vi "电流传感器测试.vi"(0 "仪器实例 out":T1, 1 "电流读取":refnum<visa-resource-name>, 2 "灵敏度":dbl, 5 "传感器缩放系数":dbl=2000.0 format="%#_13g", 9 "CAB500":enum16{"CAB500", "CAB1500"}(ring), 11 "错误输入（无错误）":errorcluster, 12 "file path (dialog if empty)":path caption="文件路径 （空时为对话框）", 14 "电压读取":bool) -> (3 "报文":string[](array[string]), 4 "仪器实例 out 2":T1, 6 "解析电流":dbl[](array[numeric]), 7 "实读电流":dbl[](array[numeric]), 8 "霍尔解析电流":dbl[](array[numeric]), 13 "十次平均":dbl[](array[numeric]), 15 "错误输出":errorcluster)   [LabVIEW 2021]
uses:
  <vilib>/Utility/file.llb/Read Delimited Spreadsheet (DBL).vi
  <instrlib>/Keithley DMM6500 DAQ6500 Series/Keithley DMM6500 DAQ6500 Series.lvlib
  <instrlib>/Keithley 27XX/Keithley 27XX.lvlib
  <vilib>/regexp/Match Regular Expression.xnode
  <instrlib>/Keithley DMM6500 DAQ6500 Series/Public/Data/Read (Single Point).vi
  <instrlib>/Keithley 27XX/Public/Data/Read Single Point.vi
panel:
  in  "仪器实例 out 4":T1
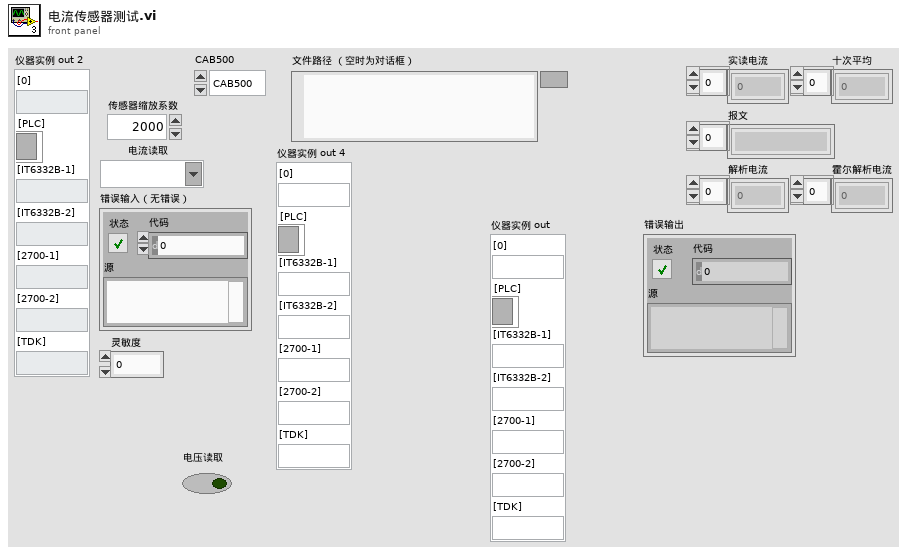
[diagram p1: front panel]
types:
  T1 = typedef "仪器实例.ctl" = cluster{"[0]":string, "[PLC]":refnum<k24>, "[IT6332B-1]":string, "[IT6332B-2]":string, "[2700-1]":string, "[2700-2]":string, "[TDK]":string}
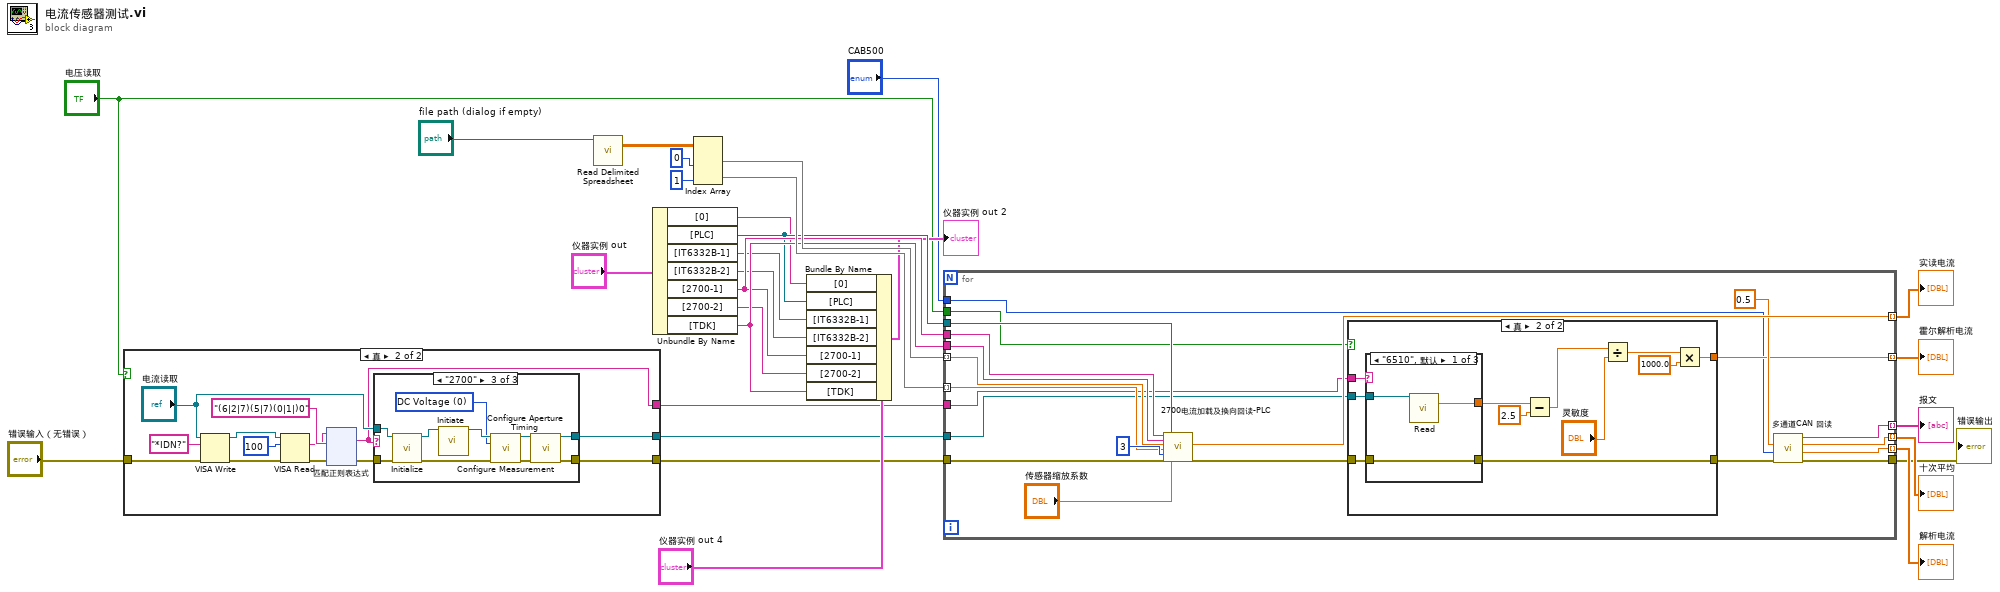
[diagram p0: block diagram]
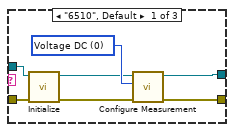
[diagram p3: hidden frame]
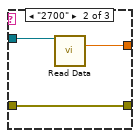
[diagram p6: hidden frame]
diagram:
  n1 = case shown="真" "电压读取" {
    tunnel: "错误输入（无错误）" -> [w29 w33]
    tunnel: [w29 w32] -> w8
    tunnel: [_ w31] -> w7
    tunnel: [_ w30] -> w6
    frame False {
    }
    frame True {
      n2 = VISA Write(VISA resource name="电流读取", write buffer="*IDN?" ("写入缓冲区"), error in (no error)=w33) -> (VISA resource name out=w40:refnum<visa-resource-name>, error out=w41:errorcluster)  [unwired: 1 out]
      n3 = VISA Read(VISA resource name=w40, byte count=u32 100 ("字节总数"), error in (no error)=w41) -> (read buffer=w37:string, error out=w36:errorcluster)  [unwired: 2 out]
      n4 = xnode "匹配正则表达式"("输入字符串"=w37, "正则表达式"="(6|2|7)(5|7)(0|1|)0", "错误输入"=w36) -> ("所有匹配"=w31:string, "错误输出"=w34:errorcluster)  [unwired: 3 in, 3 out]
      n5 = case shown="\"2700\"" w31 {
        tunnel: "电流读取" -> [w165 _ w176]
        tunnel: w34 -> [w162 _ w171]
        tunnel: [w161 _ w170] -> w30
        tunnel: [w160 _ w167] -> w32
        frame "6510", Default {
          w166 = 0 items=["Voltage DC", "Voltage AC", "Current DC", "Current AC", "Resistance", "4-wire Resistance", "Diode", "Capacitance", "Temperature", "Continuity", "Frequency", "Period", "Voltage Ratio", "Voltage", "Current"] ("Function (0: Voltage DC)")
          n6 = call <instrlib>:"Initialize.vi"("error in (no error)"=w162, "VISA resource name"=w165) -> ("error out"=w163:errorcluster, "VISA resource name out"=w164:refnum<visa-resource-name>)  [unwired: 8 in]
          n7 = call <instrlib>:"Configure Measurement.vi"("error in (no error)"=w163, "Function (0: Voltage DC)"=w166, "VISA resource name"=w164) -> ("error out"=w160:errorcluster, "VISA resource name out"=w161:refnum<visa-resource-name>)  [unwired: 7 in]
        }
        frame "7510" {
        }
        frame "2700" {
          w172 = u16 0 items=["DC Voltage", "AC Voltage", "DC Current", "AC Current", "Resistance", "Four-Wire Resistance", "Temperature", "Frequency", "Period", "Continuity"] ("Function (0: DC Voltage)")
          n8 = call <instrlib>:"Initialize.vi"("VISA resource name"=w176, "error in (no error)"=w171) -> ("VISA resource name out"=w175:refnum<visa-resource-name>, "error out"=w168:errorcluster)  [unwired: 12 in]
          n9 = call <instrlib>:"Initiate.vi"("VISA resource name"=w175) -> ("VISA resource name out"=w174:refnum<visa-resource-name>)  [unwired: 13 in, 1 out]
          n10 = call <instrlib>:"Configure Measurement.vi"("VISA resource name"=w174, "Function (0: DC Voltage)"=w172, "error in (no error)"=w168) -> ("VISA resource name out"=w173:refnum<visa-resource-name>, "error out"=w169:errorcluster)  [unwired: 11 in]
          n11 = call <instrlib>:"Configure Aperture Timing.vi"("VISA resource name"=w173, "error in (no error)"=w169) -> ("VISA resource name out"=w170:refnum<visa-resource-name>, "error out"=w167:errorcluster)  [unwired: 12 in]
        }
      }
    }
  }
  n12 = call-poly <vilib>:"Read Delimited Spreadsheet.vi"("file path (dialog if empty)"="file path (dialog if empty)") -> ("all rows"=w27:dbl[][])  [unwired: 9 in, 5 out]
  n13 = Unbundle By Name("仪器实例 out") -> ("[0]"=w11:string, "[PLC]"=w12:refnum<k24>, "[IT6332B-1]"=w13:string, "[IT6332B-2]"=w14:string, "[2700-1]"=w15:string, "[2700-2]"=w16:string, "[TDK]"=w17:string)
  n14 = Index Array(array=w27, index (col) #1=0 ("禁用的索引 (列)"), index (col) #2=1 ("索引 (列)")) -> (element #1=w25:dbl[], element #2=w24:dbl[])  [unwired: 2 in]
  n15 = Bundle By Name(cluster="仪器实例 out 4", "[0]"=w11, "[PLC]"=w12, "[IT6332B-1]"=w13, "[IT6332B-2]"=w14, "[2700-1]"=w15, "[2700-2]"=w16, "[TDK]"=w17) -> (→"仪器实例 out 2":T1)
  n16 = for {
    tunnel: w17 -> [w191]
    tunnel: w8 -> [w197]
    tunnel: [w189] -> w1
    tunnel: [w195] -> w22 mode=indexing
    tunnel: w25 -> [w194] mode=indexing
    tunnel: w24 -> [w193] mode=indexing
    tunnel: w15 -> [w192]
    tunnel: [w188] -> w21 mode=indexing
    tunnel: [w186] -> w20 mode=indexing
    tunnel: [w185] -> w19 mode=indexing
    tunnel: w12 -> [w184]
    tunnel: w7 -> [w183]
    tunnel: w6 -> [w182]
    tunnel: [w179] -> w5 mode=indexing
    tunnel: "电压读取" -> [w178]
    tunnel: "CAB500" -> [w177]
    n17 = call "2700电流加载及换向回读-PLC.vi"("6510 in"=w192, "TDK in"=w191, "输入电流"=w194, "Delay Time (s)"=w193, "电源台数"=u8 3, "error in"=w197, "引用输出"=w184, "y"="传感器缩放系数") -> ("实际电流"=w195:dbl, "error out"=w181:errorcluster)  [unwired: 8 in, 2 out]
    n18 = case shown="真" w178 {
      tunnel: w183 -> [_ w209]
      tunnel: w182 -> [_ w208]
      tunnel: w181 -> [w198 w207]
      tunnel: [w198 w206] -> w180
      tunnel: [_ w199] -> w179
      frame False {
      }
      frame True {
        n19 = case shown="\"6510\", 默认" w209 {
          tunnel: w208 -> [w212 w215 _]
          tunnel: w207 -> [w211 w214 w216]
          tunnel: [w211 w214 w216] -> w206
          tunnel: [w210 w213 _] -> w205
          frame "6510", Default {
            n20 = call-poly <instrlib>:"Read.vi"("VISA resource name"=w212) -> ("Measurement"=w210:dbl)  [unwired: 12 in, 2 out]
          }
          frame "2700" {
            n21 = call-poly <instrlib>:"Read Data.vi"("VISA resource name"=w215) -> ("Measurement Data"=w213:dbl)  [unwired: 12 in, 2 out]
          }
          frame "7510" {
          }
        }
        n22 = Subtract(x=w205, y=2.5) -> (x-y=w203:dbl)
        n23 = Divide(x=w203, y="灵敏度") -> (x/y=w201:dbl)
        n24 = Multiply(x=w201, y=1000.0) -> (x*y=w199:dbl)
      }
    }
    n25 = call "多通道CAN 回读.vi"("错误输入（无错误）"=w180, "枚举"=w177, "Delay Time (s)"=0.5) -> ("错误输出"=w189:errorcluster, "解析电流"=w185:dbl, "十次平均"=w186:dbl, "报文"=w188:string)  [unwired: 5 in]
  }
  "实读电流" <- w22
  "报文" <- w21
  "十次平均" <- w20
  "解析电流" <- w19
  "霍尔解析电流" <- w5
  "错误输出" <- w1
